vi "Open_LEDs.vi"() -> (0 "error out":errorcluster, 3 "RelayDevRef":T3={"DevStatus"={"status"=FALSE, "code"=0, "source"=""}, "Relay Channel"=enum."Invalid", "Digital Module"=enum."Digital Module 1", "Relay Direction"=enum."Both directions"})   [LabVIEW 2012]
uses:
  <vilib>/Rock Robotics/WPI/Relay/WPI_RelayDevRef.ctl
  <vilib>/Rock Robotics/SystemInterfaces/DIO/FPGA_DIORelayChannel.ctl
  <vilib>/Rock Robotics/SystemInterfaces/Typedef/FPGA_TypedefDigitalModule.ctl
  <vilib>/Rock Robotics/WPI/Relay/WPI_RelayDirection.ctl
panel:
  in  "Digital Module":T1
  in  "Relay Channel":T2=enum."Relay 4"
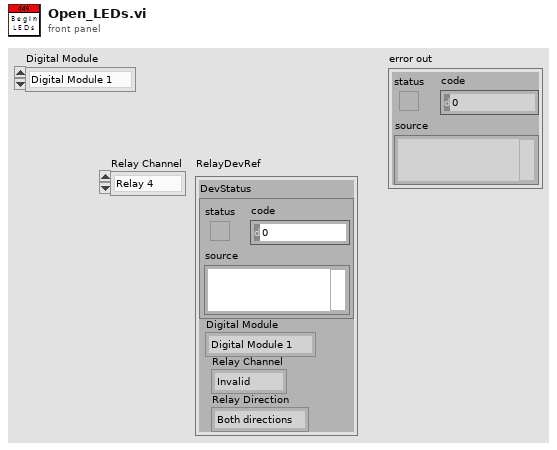
[diagram p1: front panel]
types:
  T1 = typedef "FPGA_TypedefDigitalModule.ctl" = enum16{"Digital Module 1", "Digital Module 2"}
  T2 = typedef "FPGA_DIORelayChannel.ctl" = enum8{"Relay 1", "Relay 2", "Relay 3", "Relay 4", "Relay 5", "Relay 6", "Relay 7", "Relay 8", "Invalid"}
  T3 = typedef "WPI_RelayDevRef.ctl" = cluster{"DevStatus":errorcluster, "Relay Channel":T2, "Digital Module":T1, "Relay Direction":T4}
  T4 = typedef "WPI_RelayDirection.ctl" = enum16{"Both directions", "Forward only", "Reverse only"}
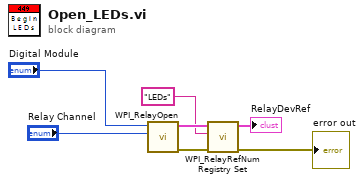
[diagram p0: block diagram]
diagram:
  n1 = call <vilib>:"WPI_RelayOpen.vi"("Relay Channel"="Relay Channel", "Digital Module (Module 1)"="Digital Module") -> ("error out"=w7:errorcluster, "RelayDevRef"=w6:T3)  [unwired: 8 in]
  n2 = call <vilib>:"WPI_RelayRefNum Registry Set.vi"("error in (no error)"=w7, "refnum name"="LEDs", "RelayDevRef"=w6) -> ("error out"=→"error out":errorcluster, "RelayDevRef"=→"RelayDevRef":T3)  [unwired: 7 in]
